vi "Night Day (SubVI).vi"(1 "To This (24HR)":i32, 2 "From This (24 HR)":i32) -> (0 "Time (CurrentTime-B/W-Range?Night:Day)":string)   [LabVIEW 2015]
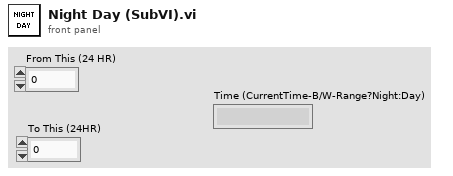
[diagram p1: front panel]
types:
  T1 = typedef "LVDateTimeRec.ctl" = cluster{"fractional second":dbl, "second":i32, "minute":i32, "hour":i32, "day of month":i32, "month":i32, "year":i32, "day of week":i32, "day of year":i32, "DST":i32}
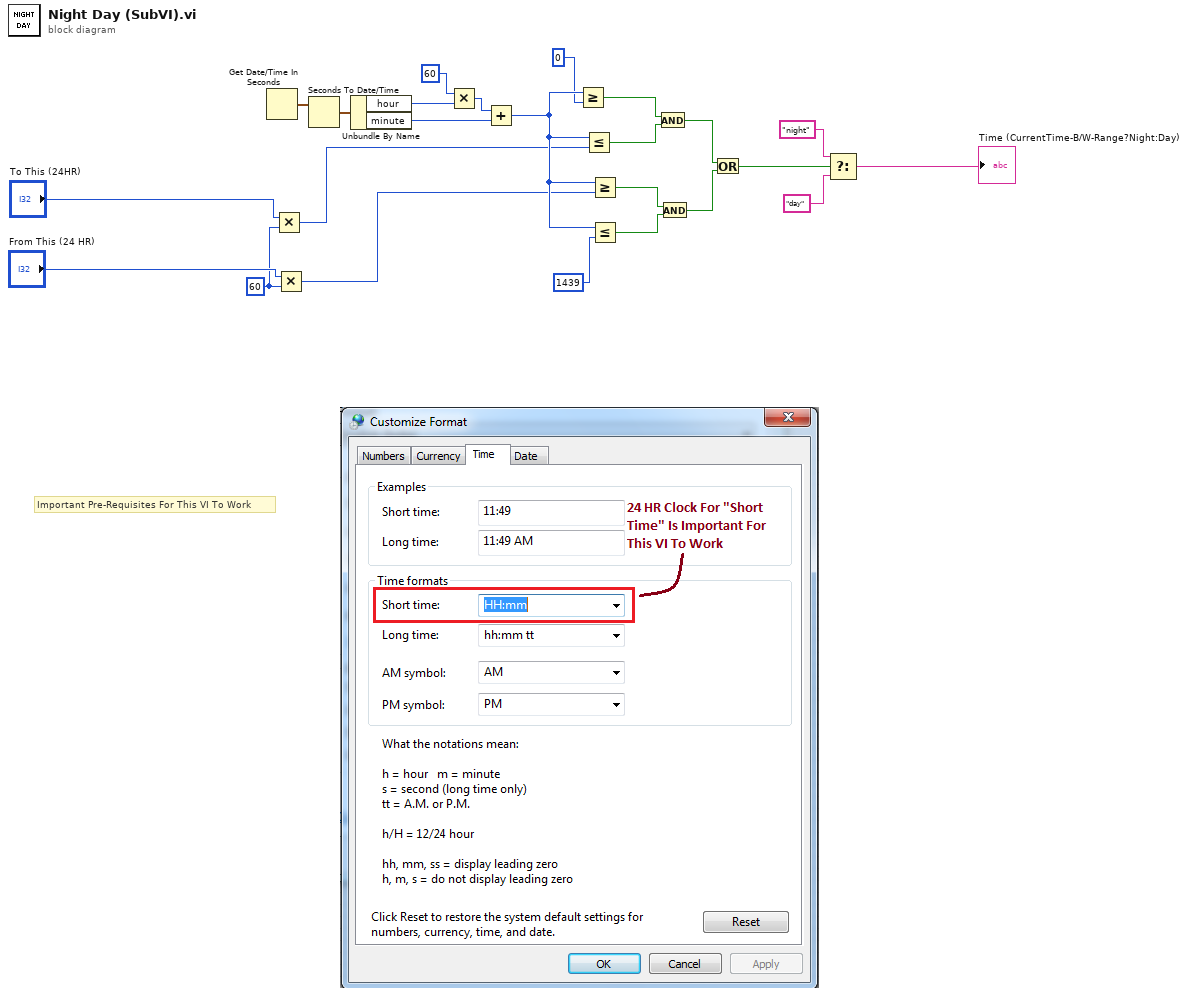
[diagram p0: block diagram]
diagram:
  w9 = 60 ("y")
  # "Important Pre-Requisites For This VI To Work"
  n1 = Get Date/Time In Seconds() -> (seconds since 1Jan1904=w13:timestamp)
  n2 = Multiply(x="To This (24HR)", y=w9) -> (x*y=w8:i32)
  n3 = Multiply(x="From This (24 HR)", y=w9) -> (x*y=w11:i32)
  n4 = Seconds To Date/Time(time stamp (now)=w13) -> (date time rec=w14:T1)  [unwired: 1 in]
  n5 = Unbundle By Name(w14) -> ("hour"=w15:i32, "minute"=w18:i32)
  n6 = Multiply(x=60, y=w15) -> (x*y=w17:i32)
  n7 = Add(x=w17, y=w18) -> (x+y=w20:i32)
  n8 = Greater Or Equal?(x=w20, y=0) -> (x >= y?=w5:bool)
  n9 = Less Or Equal?(x=w20, y=w8) -> (x <= y?=w4:bool)
  n10 = Greater Or Equal?(x=w20, y=w11) -> (x >= y?=w6:bool)
  n11 = Less Or Equal?(x=w20, y=1439) -> (x <= y?=w7:bool)
  n12 = And(x=w5, y=w4) -> (x .and. y?=w3:bool)
  n13 = And(x=w6, y=w7) -> (x .and. y?=w2:bool)
  n14 = Or(x=w3, y=w2) -> (x .or. y?=w1:bool)
  n15 = Select(t="night", s=w1, f="day") -> (s? t:f=→"Time (CurrentTime-B/W-Range?Night:Day)":string)
